vi "Unequal_Safe_VLIWarray.vi"(5 "VLIW Array x":T1(array[cluster]), 9 "VLIW Array y":T1(array[cluster])) -> (8 "Diff?":bool, 14 "Diff? array":bool[](array[boolean]))   [LabVIEW 2013]
doc: "Assesses x not equal to y?, up to length of x. The output 'which diff?' always matches the length of x. Additionally, 'diff?' is provided for convenience as the array-OR for a simple boolean indicating at lease one difference."
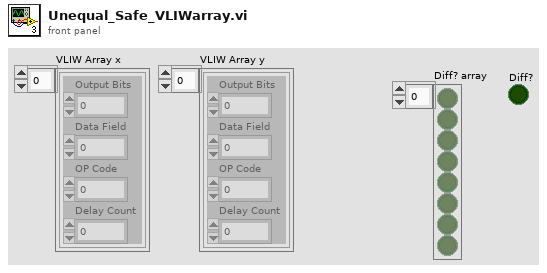
[diagram p1: front panel]
types:
  T1 = cluster{"Output Bits":u32, "Data Field":u32, "OP Code":u8, "Delay Count":u64}[]
  T2 = cluster{"Output Bits":u32, "Data Field":u32, "OP Code":u8, "Delay Count":u64}
  T3 = cluster{"Output Bits":bool, "Data Field":bool, "OP Code":bool, "Delay Count":bool}
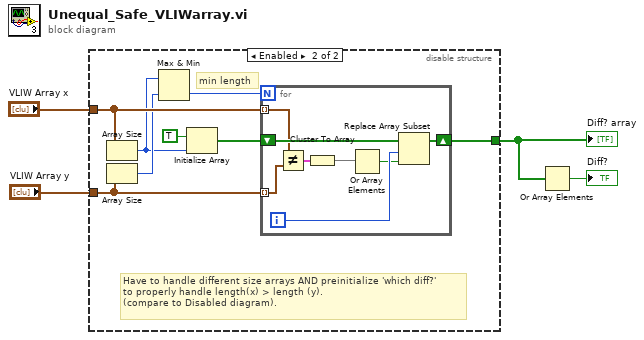
[diagram p0: block diagram]
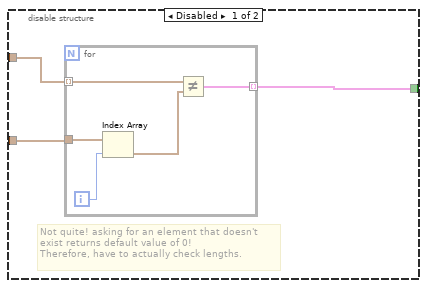
[diagram p2: hidden frame]
diagram:
  n1 = disable-structure shown="Enabled" {
    disable-tunnel: "VLIW Array x" -> [w7 w17]
    disable-tunnel: "VLIW Array y" -> [w6 w18]
    disable-tunnel: [w5 w13] -> w4
    frame Disabled {
      # "Not quite! asking for an element that doesn't \nexist returns default value of 0!\nTherefore, have to actually check lengths."
      n2 = for {
        tunnel: w7 -> [w10] mode=indexing
        tunnel: w6 -> [w12]
        tunnel: [w8] -> w5 mode=indexing
        i -> [w11]
        n3 = Index Array(array=w12, index=w11) -> (element=w9:T2)
        n4 = Not Equal?(x=w10, y=w9) -> (x != y?=w8:T3)
      }
    }
    frame Enabled {
      # "Have to handle different size arrays AND preinitialize 'which diff?'\nto properly handle length(x) > length (y).\n(compare to Disabled diagram)."
      # "min length"
      n5 = Array Size(array=w17) -> (size(s)=w15:i32)
      n6 = Array Size(array=w18) -> (size(s)=w16:i32)
      n7 = Max & Min(x=w15, y=w16) -> (min(x,y)=w14:i32)  [unwired: 1 out]
      n8 = Initialize Array(TRUE, w15) -> (w19:bool[])
      n9 = for {
        N: w14 -> [_]
        shift-right: [w27] -> w13
        shift-left: w19 -> [w28]
        tunnel: w18 -> [w25] mode=indexing
        tunnel: w17 -> [w26] mode=indexing
        i -> [w24]
        n10 = Not Equal?(x=w26, y=w25) -> (x != y?=w23:T3)
        n11 = Cluster To Array(cluster=w23) -> (array=w21:bool[])
        n12 = Or Array Elements(Boolean array=w21) -> (logical OR=w22:bool)
        n13 = Replace Array Subset(array=w28, new element=w22, index=w24) -> (w27:bool[])
      }
    }
  }
  "Diff? array" <- w4
  n14 = Or Array Elements(Boolean array=w4) -> (logical OR=→"Diff?":bool)
